vi "Температурная система.vi"() -> ()   [LabVIEW 2017]
doc: "This VI is an exercise in the LabVIEW Basics I course.\n\nYou will build the diagram for this VI so that it runs as a user-driven interface. When the user presses a button, then the appropriate subVI will open. You will be modifying the SubVI Node Setup of the subVIs and the VI Properties of this VI."
panel:
  in  "stop":bool
  in  "Вывод записанной\nтемпературы":bool
  in  "Вывод и запись \nтемпературы":bool
  in  "Вывод\nтемпературы":bool
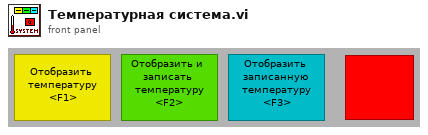
[diagram p1: front panel]
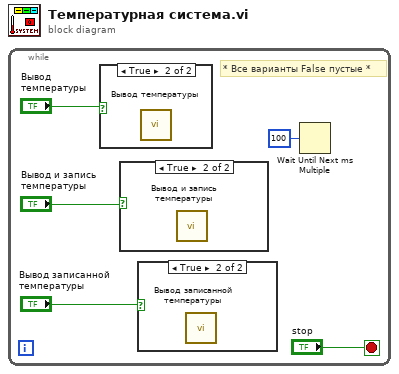
[diagram p0: block diagram]
diagram:
  n1 = while {
    stop <- "stop" stop-if-true
    # "* Все варианты False пустые *"
    n2 = case shown="True" "Вывод\nтемпературы" {
      frame False {
      }
      frame True {
        n3 = call "Вывод температуры.vi"() -> ()  [unwired: 1 in]
      }
    }
    n4 = case shown="True" "Вывод и запись \nтемпературы" {
      frame False {
      }
      frame True {
        n5 = call "Вывод и запись температуры.vi"() -> ()  [unwired: 1 in]
      }
    }
    n6 = case shown="True" "Вывод записанной\nтемпературы" {
      frame False {
      }
      frame True {
        n7 = call "Вывод записанной температуры.vi"() -> ()  [unwired: 1 in]
      }
    }
    n8 = Wait Until Next ms Multiple(millisecond multiple=u32 100) -> ()  [unwired: 1 out]
  }
